vi "Read System Module ID.vi"(8 "error in (no error)":errorcluster, 11 "System Modules Factory in":refnum<class "System Modules Factory.lvclass">) -> (0 "error out":errorcluster, 2 "System Module ID":u32[](array[numeric]), 3 "System Modules Factory out":refnum<class "System Modules Factory.lvclass">)   [LabVIEW 2019, in "System Modules Factory.lvclass"]
uses:
  System Modules Factory.lvclass
  System Modules Factory.lvclass/System Modules Factory.ctl
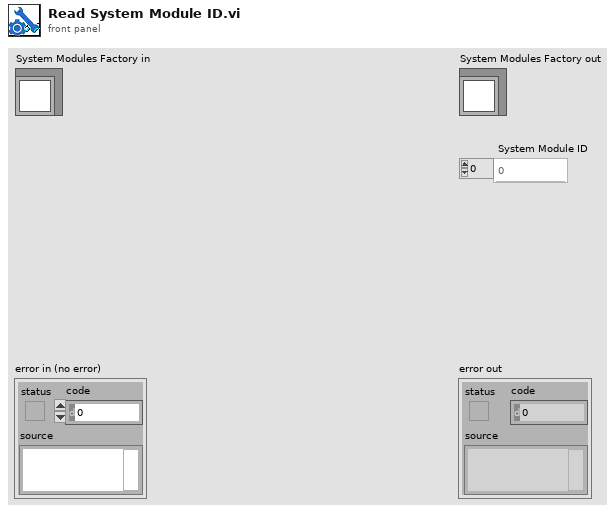
[diagram p1: front panel]
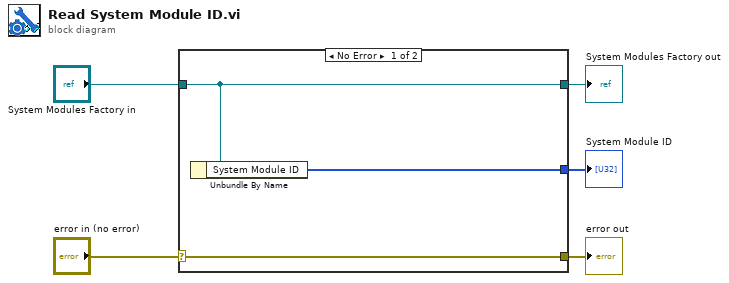
[diagram p0: block diagram]
diagram:
  n1 = case shown="No Error" "error in (no error)" {
    selector: "error in (no error)" -> [w8 w9]
    tunnel: [w8 w9] -> w4
    tunnel: [w7 w10] -> w2
    tunnel: "System Modules Factory in" -> [w7 w10]
    tunnel: [w6 _] -> w1
    frame No Error {
      n2 = Unbundle By Name(w7) -> ("System Module ID"=w6:u32[])
    }
    frame Error {
    }
  }
  "error out" <- w4
  "System Modules Factory out" <- w2
  "System Module ID" <- w1
